vi "Live window-Shortcut menus handler.vi"(11 "ItemTag":string) -> ()   [LabVIEW 2020]
uses:
  Typedefs/Left-Right enum.ctl
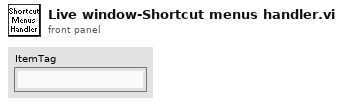
[diagram p1: front panel]
types:
  T1 = typedef "Left-Right enum.ctl" = enum16{"Right", "Left"}
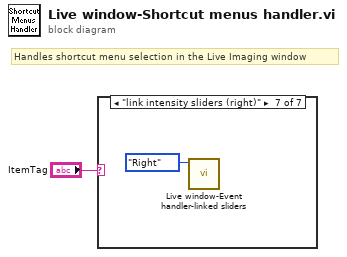
[diagram p0: block diagram]
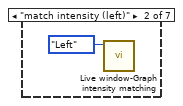
[diagram p3: hidden frame]
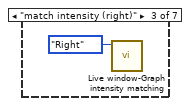
[diagram p4: hidden frame]
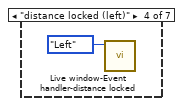
[diagram p5: hidden frame]
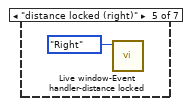
[diagram p6: hidden frame]
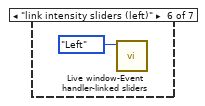
[diagram p7: hidden frame]
diagram:
  # "Handles shortcut menu selection in the Live Imaging window"
  n1 = case shown="\"link intensity sliders (right)\"" "ItemTag" {
    frame Default {
    }
    frame "match intensity (left)" {
      n2 = call "Live window-Graph intensity matching.vi"("Left/Right"=Left-Right_enum."Left") -> ()  [unwired: 10 in, 1 out]
    }
    frame "match intensity (right)" {
      n3 = call "Live window-Graph intensity matching.vi"("Left/Right"=Left-Right_enum."Right") -> ()  [unwired: 10 in, 1 out]
    }
    frame "distance locked (left)" {
      n4 = call "Live window-Event handler-distance locked.vi"("Function"=Left-Right_enum."Left") -> ()  [unwired: 11 in]
    }
    frame "distance locked (right)" {
      n5 = call "Live window-Event handler-distance locked.vi"("Function"=Left-Right_enum."Right") -> ()  [unwired: 11 in]
    }
    frame "link intensity sliders (left)" {
      n6 = call "Live window-Event handler-linked sliders.vi"("Left/Right"=Left-Right_enum."Left" ("Function")) -> ()  [unwired: 11 in]
    }
    frame "link intensity sliders (right)" {
      n7 = call "Live window-Event handler-linked sliders.vi"("Left/Right"=Left-Right_enum."Right" ("Function")) -> ()  [unwired: 11 in]
    }
  }
